vi "Parse Signal List.vi"(11 "Signal List":string[][](array[string])) -> (0 "Pins":i32[](array[numeric]), 1 "Control?":bool[](array[boolean]), 2 "Names":string[](array[string]), 3 "XOR List":string[](array[string]))   [LabVIEW 2019, in "DIG_IO.lvlib" / "DIG_IO.lvclass"]
uses:
  Library/DIG_IO.lvclass
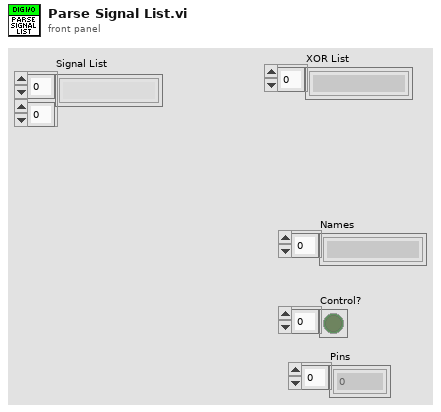
[diagram p1: front panel]
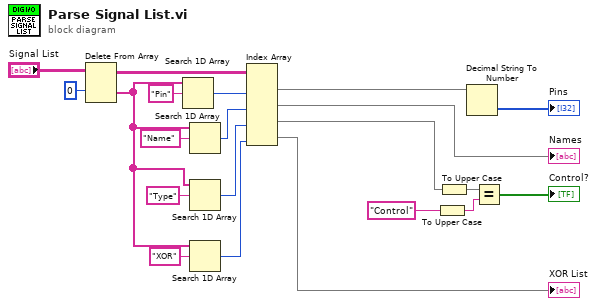
[diagram p0: block diagram]
diagram:
  n1 = Delete From Array(array="Signal List", index (row)=0) -> (deleted portion=w2:string[], array with subset deleted=w3:string[][])  [unwired: 2 in]
  n2 = Search 1D Array(1D array=w2, element="Pin") -> (index of element=w20:i32)  [unwired: 1 in]
  n3 = Search 1D Array(1D array=w2, element="Name") -> (index of element=w17:i32)  [unwired: 1 in]
  n4 = Search 1D Array(1D array=w2, element="Type") -> (index of element=w13:i32)  [unwired: 1 in]
  n5 = Search 1D Array(1D array=w2, element="XOR") -> (index of element=w7:i32)  [unwired: 1 in]
  n6 = Index Array(array=w3, index (col) #1=w20, index (col) #2=w17, index (col) #3=w13, index (col) #4=w7) -> (element #1=w19:string[], element #2=→"Names":string[], element #3=w11:string[], element #4=→"XOR List":string[])  [unwired: 4 in]
  n7 = To Upper Case(1:"Control" ("element")) -> (0:w9:string)
  n8 = To Upper Case(1:w11) -> (0:w10:string[])
  n9 = Decimal String To Number(string=w19) -> (number=→"Pins":i32[])  [unwired: 2 in, 1 out]
  n10 = Equal?(x=w10, y=w9) -> (x = y?=→"Control?":bool[])
